vi "Test AVS47B Remote Control.vi"() -> ()   [LabVIEW 2012]
doc: "Application example"
panel:
  in  "stop":bool
  in  "VISA RESOURCE":refnum<visa-resource-name>="COM4"
  # "Test AVS47B Remote Control.vi"
  # "This VI tests the AVS47B front panel LEDs and  their hardware\nregisters. Then it sets the digital reference to 0, 10, 100, 1000,\n10000 and 19000 microvolts. During this phase, display is set to \nREFERENCE. This is a complete application that can be run\nas such.\n\nNOTE: If the TS-530A is connected to the resistance bridge\nduring this test, it must also be powered.  An unpowered\nTS-530A would load the data lines excessively."
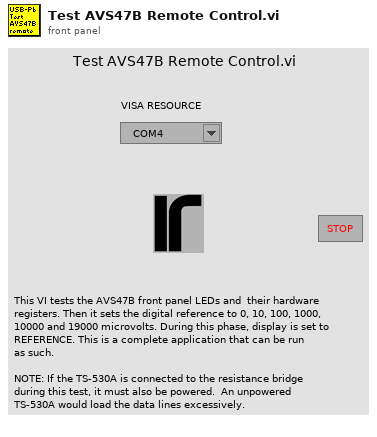
[diagram p1: front panel]
types:
  T1 = enum16{"INPUT LEDS", "CH LEDS", "RANGE LEDS", "EXC LEDS", "DISP LEDS", "REFERENCE", "FINISH"}
  T2 = cluster{"VISA RESOURCE":refnum<visa-resource-name>, "PICOBUS ADDRESS":u8, "DISABLE AL":u8, "REMOTE":u8, "INPUT":u8, "CHANNEL":u8, "RANGE":u8, "EXCITATION":u8, "DISPLAY":u8, "DIGITAL REFERENCE":u16, "SET POINT":dbl, "PROP GAIN":u8, "INTG":u8, "DERIV":u8, "POWER BIAS":u8, "POWER RANGE":u8, "INFO STRING":string, "HEATER RESISTANCE":dbl, "INTERVAL":u8, " SENSOR dR/dT":u8}
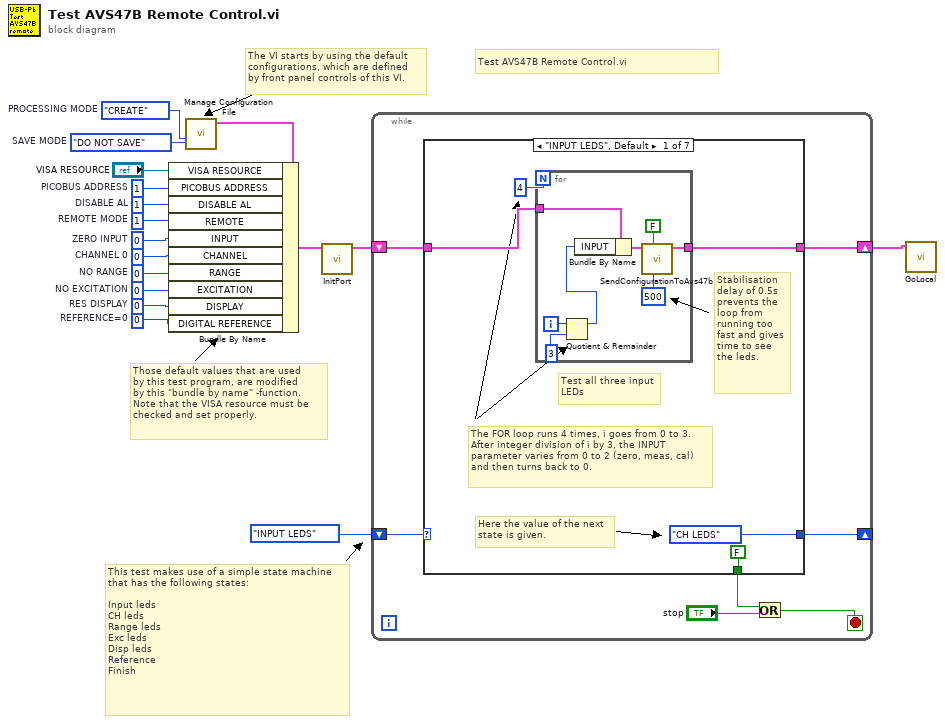
[diagram p0: block diagram]
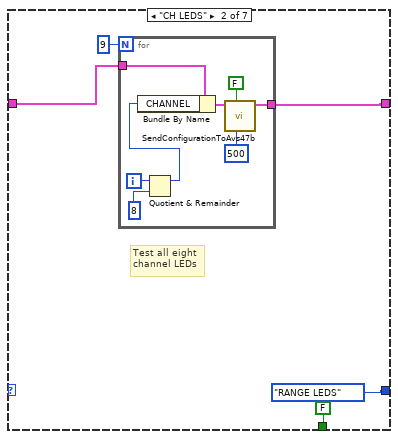
[diagram p2: hidden frame]
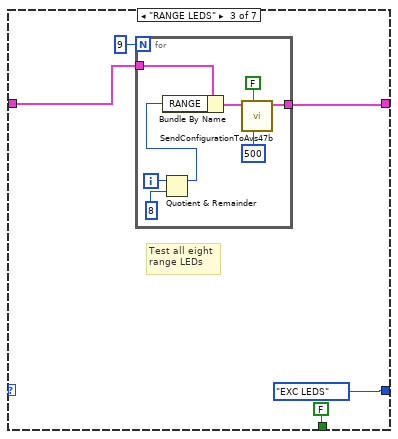
[diagram p3: hidden frame]
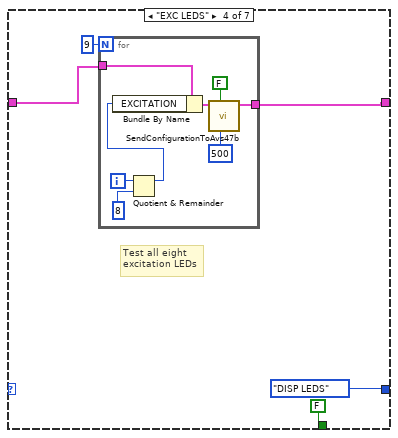
[diagram p4: hidden frame]
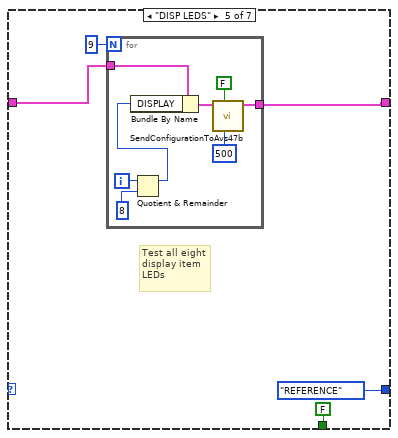
[diagram p5: hidden frame]
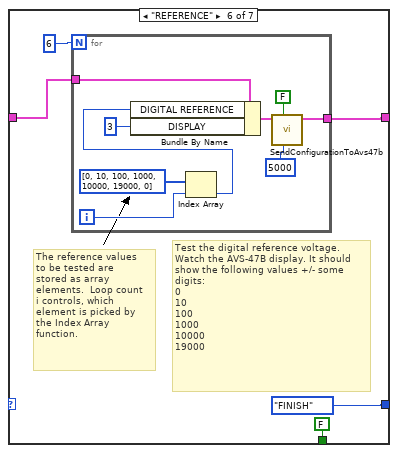
[diagram p6: hidden frame]
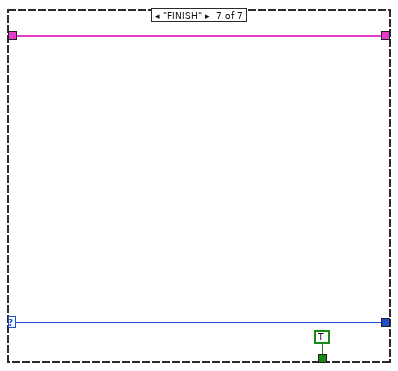
[diagram p7: hidden frame]
diagram:
  w3 = enum16{"DO NOT SAVE", "SAVE .CNF FILE"}."DO NOT SAVE"  # SAVE MODE
  w4 = enum16{"NONE", "READ", "CREATE"}."CREATE"  # PROCESSING MODE
  w6 = u8 0  # REFERENCE=0
  w7 = u8 0  # RES DISPLAY
  w8 = u8 0  # NO EXCITATION
  w9 = u8 0  # NO RANGE
  w10 = u8 0  # CHANNEL 0
  w11 = u8 0  # ZERO INPUT
  w12 = u8 1  # REMOTE MODE
  w13 = u8 1  # DISABLE AL
  w14 = u8 1  # PICOBUS ADDRESS
  # "This test makes use of a simple state machine\nthat has the following states:\n\nInput leds\nCH leds\nRange leds\nExc leds\nDisp leds\nReference\nFinish"
  # "The VI starts by using the default\nconfigurations, which are defined\nby front panel controls of this VI."
  # "Test AVS47B Remote Control.vi"
  # "Those default values that are used\nby this test program, are modified\nby this \"bundle by name\" -function. \nNote that the VISA resource must be\nchecked and set properly."
  n1 = call "Manage Configuration File.vi"("SAVE MODE"=w3, "PROCESSING MODE"=w4) -> ("CONFIGURATION CLUSTER OUT"=w16:T2)  [unwired: 9 in]
  n2 = Bundle By Name(cluster=w16, "VISA RESOURCE"="VISA RESOURCE", "PICOBUS ADDRESS"=w14, "DISABLE AL"=w13, "REMOTE"=w12, "INPUT"=w11, "CHANNEL"=w10, "RANGE"=w9, "EXCITATION"=w8, "DISPLAY"=w7, "DIGITAL REFERENCE"=w6) -> (w1:T2)
  n3 = call "InitPort.vi"("CONFIGURATION CLUSTER"=w1) -> ("UNMODIFIED CONFIGURATION CLUSTER"=w2:T2)  [unwired: 6 in, 2 out]
  n4 = while {
    shift-right: [w22] -> _
    shift-left: T1."INPUT LEDS" -> [w18]
    shift-right: [w23] -> w5
    shift-left: w2 -> [w24]
    stop <- w19 stop-if-true
    n5 = case shown="\"INPUT LEDS\", Default" w18 {
      selector: w18 -> [_ _ _ _ _ _ w104]
      tunnel: w24 -> [w28 w41 w54 w67 w80 w92 w105]
      tunnel: [w27 w40 w53 w66 w79 w93 w105] -> w23
      tunnel: [T1."CH LEDS" T1."RANGE LEDS" T1."EXC LEDS" T1."DISP LEDS" T1."REFERENCE" T1."FINISH" w104] -> w22
      tunnel: [FALSE ("x") FALSE ("x") FALSE ("x") FALSE ("x") FALSE ("x") FALSE ("x") TRUE ("x")] -> w20
      frame "INPUT LEDS", Default {
        # "Here the value of the next\nstate is given."
        # "Stabilisation\ndelay of 0.5s\nprevents the\nloop from\nrunning too\nfast and gives\ntime to see\nthe leds."
        # "The FOR loop runs 4 times, i goes from 0 to 3.\nAfter integer division of i by 3, the INPUT \nparameter varies from 0 to 2 (zero, meas, cal)\nand then turns back to 0."
        # "Test all three input\nLEDs"
        n6 = for {
          N: 4 -> [_]
          tunnel: w28 -> [w34]
          tunnel: [w30] -> w27
          i -> [w33]
          n7 = Quotient & Remainder(x=w33, y=3) -> (x-y*floor(x/y)=w31:i32)  [unwired: 1 out]
          n8 = Bundle By Name(cluster=w34, "INPUT"=w31) -> (w35:T2)
          n9 = call "SendConfigurationToAvs47b.vi"("STABILISATION DELAY (ms)"=500, "WRITE ALSO TO TS-530A"=FALSE, "CONFIGURATION CLUSTER"=w35) -> ("UNMODIFIED CONFIGURATION CLUSTER"=w30:T2)  [unwired: 5 in, 3 out]
        }
      }
      frame "CH LEDS" {
        # "Test all eight \nchannel LEDs"
        n10 = for {
          N: 9 -> [_]
          tunnel: w41 -> [w47]
          tunnel: [w43] -> w40
          i -> [w46]
          n11 = Quotient & Remainder(x=w46, y=8) -> (x-y*floor(x/y)=w44:i32)  [unwired: 1 out]
          n12 = Bundle By Name(cluster=w47, "CHANNEL"=w44) -> (w48:T2)
          n13 = call "SendConfigurationToAvs47b.vi"("STABILISATION DELAY (ms)"=500, "WRITE ALSO TO TS-530A"=FALSE, "CONFIGURATION CLUSTER"=w48) -> ("UNMODIFIED CONFIGURATION CLUSTER"=w43:T2)  [unwired: 5 in, 3 out]
        }
      }
      frame "RANGE LEDS" {
        # "Test all eight \nrange LEDs"
        n14 = for {
          N: 9 -> [_]
          tunnel: w54 -> [w60]
          tunnel: [w56] -> w53
          i -> [w59]
          n15 = Quotient & Remainder(x=w59, y=8) -> (x-y*floor(x/y)=w57:i32)  [unwired: 1 out]
          n16 = Bundle By Name(cluster=w60, "RANGE"=w57) -> (w61:T2)
          n17 = call "SendConfigurationToAvs47b.vi"("STABILISATION DELAY (ms)"=500, "WRITE ALSO TO TS-530A"=FALSE, "CONFIGURATION CLUSTER"=w61) -> ("UNMODIFIED CONFIGURATION CLUSTER"=w56:T2)  [unwired: 5 in, 3 out]
        }
      }
      frame "EXC LEDS" {
        # "Test all eight\nexcitation LEDs"
        n18 = for {
          N: 9 -> [_]
          tunnel: w67 -> [w73]
          tunnel: [w69] -> w66
          i -> [w72]
          n19 = Quotient & Remainder(x=w72, y=8) -> (x-y*floor(x/y)=w70:i32)  [unwired: 1 out]
          n20 = Bundle By Name(cluster=w73, "EXCITATION"=w70) -> (w74:T2)
          n21 = call "SendConfigurationToAvs47b.vi"("STABILISATION DELAY (ms)"=500, "WRITE ALSO TO TS-530A"=FALSE, "CONFIGURATION CLUSTER"=w74) -> ("UNMODIFIED CONFIGURATION CLUSTER"=w69:T2)  [unwired: 5 in, 3 out]
        }
      }
      frame "DISP LEDS" {
        # "Test all eight\ndisplay item\nLEDs"
        n22 = for {
          N: 9 -> [_]
          tunnel: w80 -> [w86]
          tunnel: [w82] -> w79
          i -> [w85]
          n23 = Quotient & Remainder(x=w85, y=8) -> (x-y*floor(x/y)=w83:i32)  [unwired: 1 out]
          n24 = Bundle By Name(cluster=w86, "DISPLAY"=w83) -> (w87:T2)
          n25 = call "SendConfigurationToAvs47b.vi"("STABILISATION DELAY (ms)"=500, "WRITE ALSO TO TS-530A"=FALSE, "CONFIGURATION CLUSTER"=w87) -> ("UNMODIFIED CONFIGURATION CLUSTER"=w82:T2)  [unwired: 5 in, 3 out]
        }
      }
      frame "REFERENCE" {
        # "The reference values\nto be tested are \nstored as array\nelements.  Loop count\ni controls, which \nelement is picked by\nthe Index Array\nfunction."
        # "Test the digital reference voltage.\nWatch the AVS-47B display. It should\nshow the following values +/- some\ndigits:\n0\n10\n100\n1000\n10000\n19000"
        n26 = for {
          N: 6 -> [_]
          tunnel: w92 -> [w100]
          tunnel: [w99] -> w93
          i -> [w97]
          n27 = Index Array(array=i32[] [0, 10, 100, 1000, 10000, 19000, 0], index=w97) -> (element=w96:i32)
          n28 = Bundle By Name(cluster=w100, "DIGITAL REFERENCE"=w96, "DISPLAY"=u8 3) -> (w101:T2)
          n29 = call "SendConfigurationToAvs47b.vi"("STABILISATION DELAY (ms)"=5000, "WRITE ALSO TO TS-530A"=FALSE, "CONFIGURATION CLUSTER"=w101) -> ("UNMODIFIED CONFIGURATION CLUSTER"=w99:T2)  [unwired: 5 in, 3 out]
        }
      }
      frame "FINISH" {
      }
    }
    n30 = Or(x=w20, y="stop") -> (x .or. y?=w19:bool)
  }
  n31 = call "GoLocal.vi"("CONFIGURATION CLUSTER"=w5) -> ()  [unwired: 10 in, 1 out]
